vi "ExportToXMI.vi"(0 "reference":refnum<class "Graph.lvclass">, 1 "nodeInfo":T2, 2 "edgeInfo":T1, 3 "DiagramData":string, 5 "error in (no error)":errorcluster) -> (14 "reference out":refnum<class "Graph.lvclass">, 16 "XMIText":string, 19 "error out":errorcluster)   [LabVIEW 2020, in "Graph.lvclass"]
uses:
  <resource>/Framework/Providers/Open_GDS/UML/Graph_class/Graph.lvclass
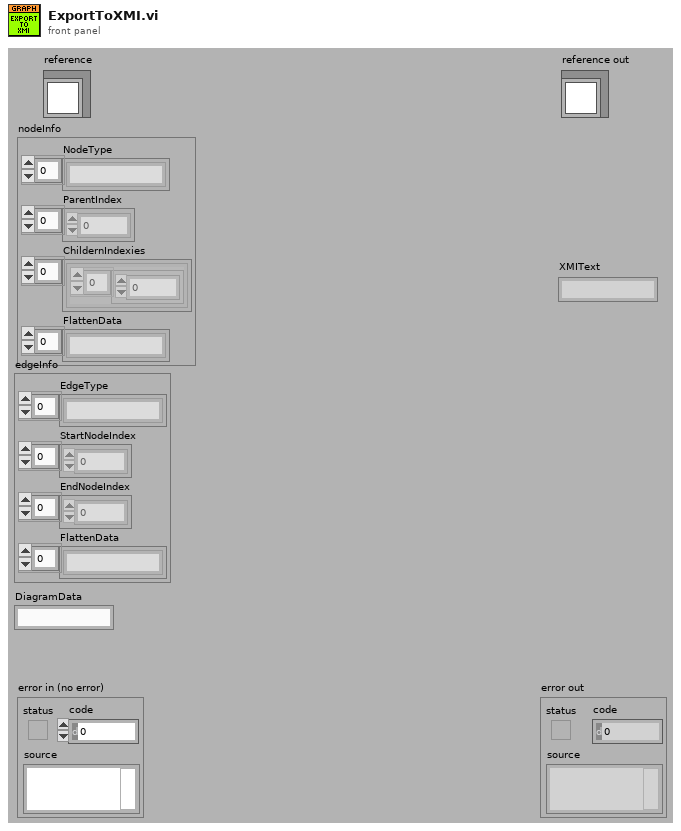
[diagram p1: front panel]
types:
  T1 = cluster{"EdgeType":string[], "StartNodeIndex":i32[], "EndNodeIndex":i32[], "FlattenData":string[]}
  T2 = cluster{"NodeType":string[], "ParentIndex":i32[], "ChildernIndexies":cluster{i32[]}[], "FlattenData":string[]}
  T3 = typedef "Graph.lvclass/ObjectAttributes.ctl" = cluster{"nodes":refnum<class "AbstractNode.lvclass">[], "edges":refnum<class "AbstractEdge.lvclass">[], "nodesToBeRemoved":refnum<class "AbstractNode.lvclass">[], "edgesToBeRemoved":refnum<class "AbstractEdge.lvclass">[], "needsLayout":bool, "LayoutNodes":refnum<class "AbstractNode.lvclass">[]}
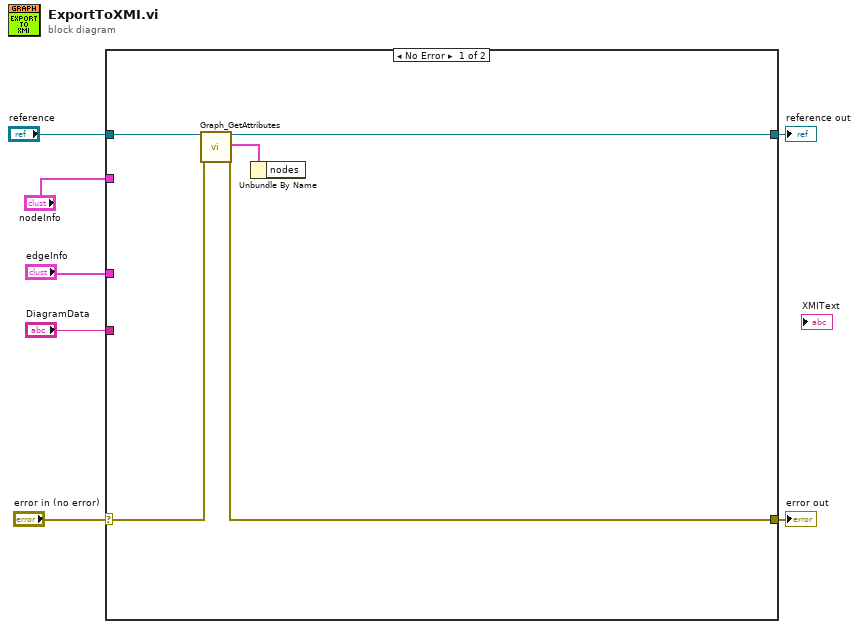
[diagram p0: block diagram]
diagram:
  n1 = case shown="No Error" "error in (no error)" {
    selector: "error in (no error)" -> [w9 w13]
    tunnel: "reference" -> [w12 w14]
    tunnel: [w11 w13] -> w6
    tunnel: [w10 w14] -> w5
    tunnel: "nodeInfo" -> [_ _]
    tunnel: "edgeInfo" -> [_ _]
    tunnel: "DiagramData" -> [_ _]
    frame No Error {
      n2 = call <resource>:"Graph_GetAttributes.vi"("reference in"=w12, "error in (no error)"=w9) -> ("reference out"=w10:refnum<class "Graph.lvclass">, "Data"=w8:T3, "error out"=w11:errorcluster)  [unwired: 1 in, 14 out]
      n3 = Unbundle By Name(w8) -> ()  [unwired: 1 out]
    }
    frame Error {
    }
  }
  "reference out" <- w5
  "error out" <- w6
